vi "set feedback settings.vi"(8 "error in (no error)":errorcluster, 10 "feedback_settings":T1, 11 "id":i32) -> (0 "error out":errorcluster, 3 "function return":i32)   [LabVIEW 2012, in "libximc.lvlib"]
doc: "result_t XIMC_API set_feedback_settings (device_t id, const feedback_settings_t* feedback_settings);"
uses:
  libximc.lvlib
  libximc.dll
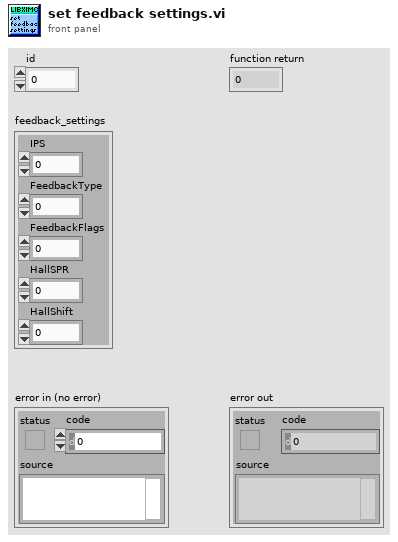
[diagram p1: front panel]
types:
  T1 = cluster{"IPS":u32, "FeedbackType":u32, "FeedbackFlags":u32, "HallSPR":u32, "HallShift":i32}
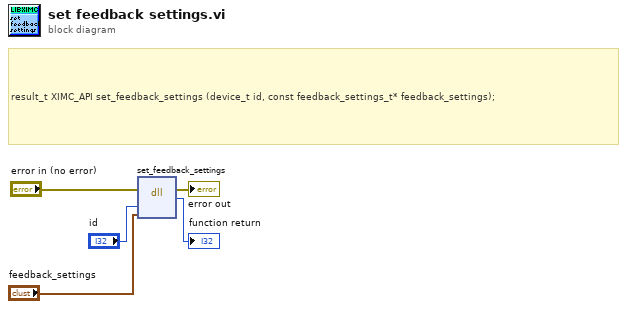
[diagram p0: block diagram]
diagram:
  # "result_t XIMC_API set_feedback_settings (device_t id, const feedback_settings_t* feedback_settings);"
  n1 = dll-call lib="C:/Users/Vasily/Att_examples/LabVIEW_example/libximc.*" fn="set_feedback_settings"(error in="error in (no error)", "id"="id", "feedback_settings"="feedback_settings") -> (error out=→"error out":errorcluster, →"function return":i32)  [unwired: 4 in, 1 out]
